vi "qSPA_String.vi"(0 "System no.":i32=1 min=1 max=4 step=1, 2 "Axes to query":string[](array[string]), 3 "Parameter no.":i32[](array[numeric]), 5 "error in":errorcluster) -> (14 "Parameter string":string[](array[string]), 19 "error out":errorcluster)   [LabVIEW 2026]
doc: "Returns parameter strings for queried axes and parameter numbers. See SPA_String.vi for available parameter numbers. For parameter numbers which output a numerical value use SPA?.vi.\nOld VI - please use SPA?.vi instead.\n\nC-843, C-843.PM, C-865: the following parameter number is valid:\n60: stage name (maximum 14 characters)"
uses:
  Communication/Global1.vi
panel:
  # "Returns parameter strings for queried axes and parameter numbers.\nOld VI - please use SPA?.vi instead."
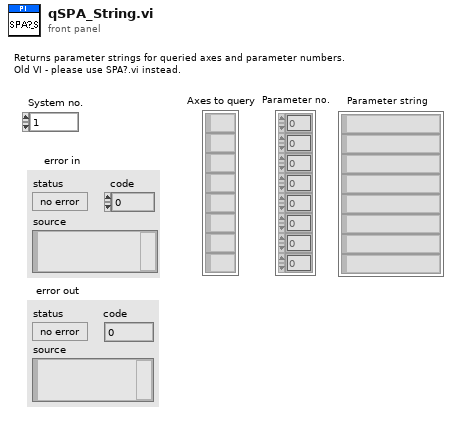
[diagram p1: front panel]
types:
  T1 = enum16{"Disable error check", "Force error check", "Use global settings"}
  T2 = typedef "Syntax.ctl" = enum16{"GCS 1.0", "GCS 2.0", "GCS 3.0"}
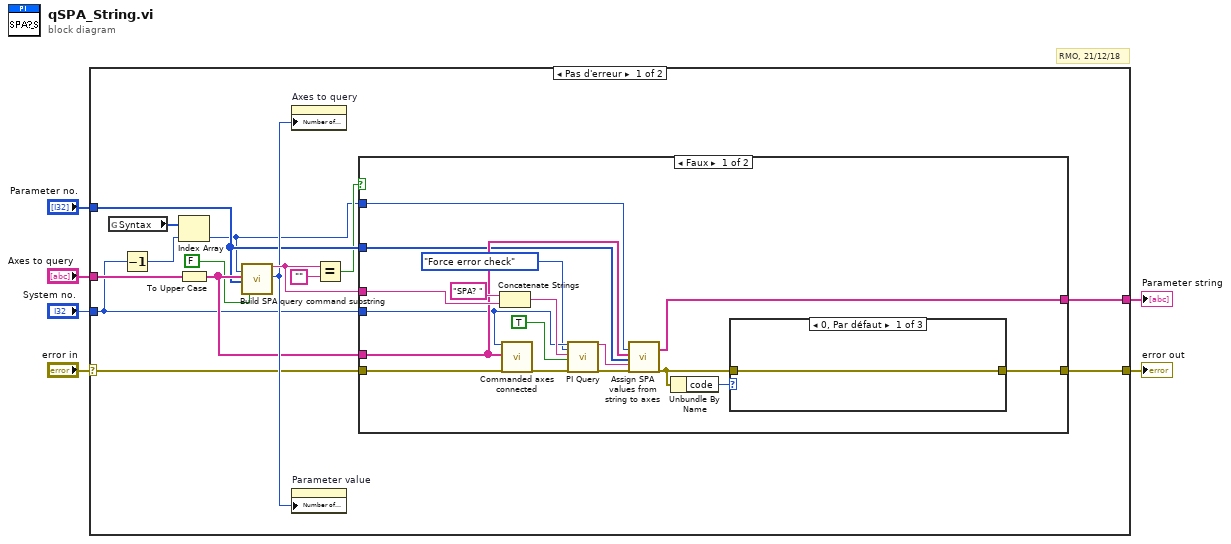
[diagram p0: block diagram]
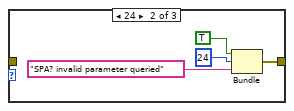
[diagram p2: hidden frame]
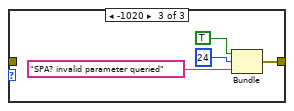
[diagram p3: hidden frame]
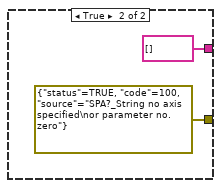
[diagram p4: hidden frame]
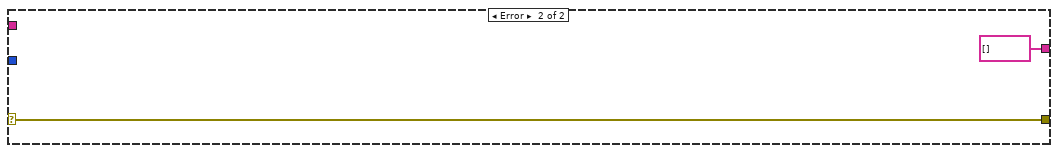
[diagram p5: hidden frame]
diagram:
  # "RMO, 21/12/18"
  n1 = case shown="Pas d'erreur" "error in" {
    selector: "error in" -> [w7 w50]
    tunnel: "Axes to query" -> [w21 _]
    tunnel: "System no." -> [w8 _]
    tunnel: "Parameter no." -> [w16 _]
    tunnel: [w15 w50] -> w3
    tunnel: [w13 string[] [] ("Parameter strings")] -> w2
    frame No Error {
      n2 = global read "Global1.vi" "Syntax"() -> (w11:T2[])
      n3 = Decrement(x=w8) -> (x-1=w12:i32)
      n4 = Index Array(array=w11, index=w12) -> (element=w10:T2)
      n5 = To Upper Case(1:w21) -> (0:w17:string[])
      n6 = call "Build SPA query command substring.vi"("Syntax"=w10, "Axes to query"=w17, "Parameter number"=w16, "Parameter no. format \n(Decimal: FALSE)"=FALSE ("Parameter no. format \n(Decimal: FALSE)")) -> ("Command substring"=w19:string, "Number of rows"=w18:u32)  [unwired: 3 in, 11 out]
      n7 = property on="Axes to query" class="Tabl (strict)"("Number of Rows"=w18) -> ()  [unwired: 2 in, 2 out]
      n8 = property on="Parameter value" class="Tabl (strict)"("Number of Rows"=w18) -> ()  [unwired: 2 in, 2 out]
      n9 = Equal?(x=w19, y="" ("x")) -> (x = y?=w14:bool)
      n10 = case shown="Faux" w14 {
        tunnel: w7 -> [w35 _]
        tunnel: w19 -> [w34 _]
        tunnel: w17 -> [w33 _]
        tunnel: w8 -> [w29 _]
        tunnel: w16 -> [w32 _]
        tunnel: [w25 errorcluster {"status"=TRUE, "code"=100, "source"="SPA?_String no axis specified\nor parameter no. zero"} ("error out")] -> w15
        tunnel: [w30 string[] [] ("Parameter strings")] -> w13
        tunnel: w10 -> [w28 _]
        frame False {
          n11 = Concatenate Strings("SPA? ", w34) -> (w36:string)
          n12 = call "Commanded axes connected.vi"("System no."=w29, "Commanded axes"=w33, "error in"=w35) -> ("error out"=w31:errorcluster)  [unwired: 1 in, 15 out]
          n13 = call "PI Query.vi"("System no."=w29, "Error check settings"=T1."Force error check", "String to send"=w36, "Attach termination char.?"=TRUE ("Attach Linefeed?"), "error in"=w31) -> ("String read"=w23:string, "error out"=w27:errorcluster)  [unwired: 2 in, 11 out]
          n14 = call "Assign SPA values from string to axes.vi"("Syntax"=w28, "Queried axes"=w33, "Parameter no."=w32, "Input string"=w23, "error in"=w27) -> ("Parameter strings"=w30:string[], "error out"=w24:errorcluster)  [unwired: 3 in, 10 out]
          n15 = Unbundle By Name(w24) -> ("code"=w26:i32)
          n16 = case shown="0, Par défaut" w26 {
            tunnel: [w39 w40 w44] -> w25
            tunnel: w24 -> [w39 _ _]
            frame 0, Default {
            }
            frame 24 {
              n17 = Bundle(TRUE, 24, "SPA? invalid parameter queried") -> (w40:errorcluster)  [unwired: 1 out]
            }
            frame -1020 {
              n18 = Bundle(TRUE, 24, "SPA? invalid parameter queried") -> (w44:errorcluster)  [unwired: 1 out]
            }
          }
        }
        frame True {
        }
      }
    }
    frame Error {
    }
  }
  "error out" <- w3
  "Parameter string" <- w2
